vi "DB- Part setting.vi"(5 "string":string="Where partno='", 6 "Enum":T2(ring), 7 "Data Insert":variant, 8 "error in (no error)":errorcluster, 9 "columnsName":string[](array[string]), 10 "Model Name":string, 11 "connection reference":T1) -> (0 "error out":errorcluster, 2 "Data Read":variant[][](array[variant]), 3 "Refnum out":T1)   [LabVIEW 2015]
uses:
  <vilib>/addons/database/Connection.llb/Conn ObjectReference.ctl
  <vilib>/addons/database/NI_Database_API.lvlib
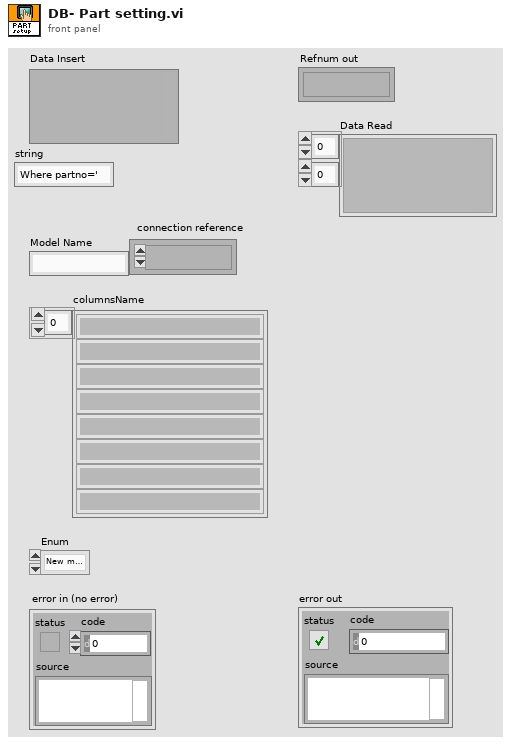
[diagram p1: front panel]
types:
  T1 = typedef "NI_Database_API.lvlib/Conn ObjectReference.ctl" = refnum<k1>
  T2 = enum16{"New model Create", "Update", "DB-Read by condition", "DB-Read", "Delete"}
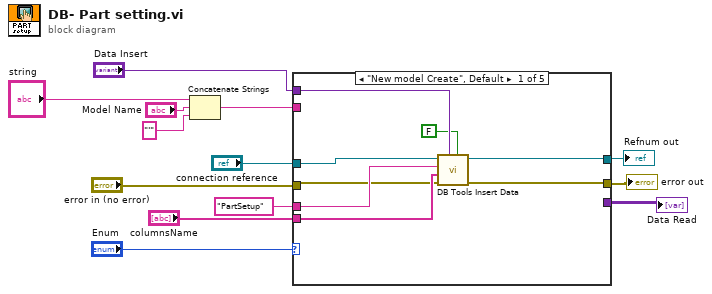
[diagram p0: block diagram]
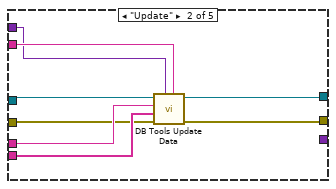
[diagram p2: hidden frame]
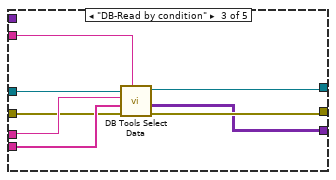
[diagram p3: hidden frame]
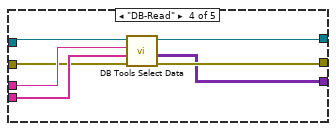
[diagram p4: hidden frame]
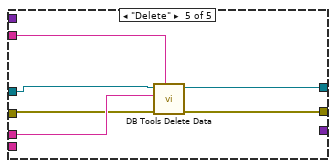
[diagram p5: hidden frame]
diagram:
  n1 = Concatenate Strings("string", "Model Name", "'" ("string")) -> (w9:string)
  n2 = case shown="\"New model Create\", Default" "Enum" {
    tunnel: [w21 w29 w34 w44 w50] -> w4
    tunnel: [w20 w28 w33 w43 w49] -> w5
    tunnel: w9 -> [_ w27 w37 _ w48]
    tunnel: "columnsName" -> [w19 w26 w36 w40 _]
    tunnel: "PartSetup" ("table") -> [w18 w25 w35 w41 w47]
    tunnel: "Data Insert" -> [w17 w24 _ _ _]
    tunnel: [_ _ w32 w42 _] -> w13
    tunnel: "connection reference" -> [w16 w23 w31 w39 w46]
    tunnel: "error in (no error)" -> [w15 w22 w30 w38 w45]
    frame "New model Create", Default {
      n3 = call <vilib>:"DB Tools Insert Data.vi"("create table? (F)"=FALSE, "data"=w17, "error in (no error)"=w15, "columns"=w19, "table"=w18, "connection reference"=w16) -> ("error out"=w20:errorcluster, "connection reference out"=w21:T1)  [unwired: 4 in]
    }
    frame "Update" {
      n4 = call <vilib>:"DB Tools Update Data.vi"("condition"=w27, "data"=w24, "error in (no error)"=w22, "columns"=w26, "table"=w25, "connection reference"=w23) -> ("error out"=w28:errorcluster, "connection reference out"=w29:T1)  [unwired: 4 in]
    }
    frame "DB-Read by condition" {
      n5 = call <vilib>:"DB Tools Select Data.vi"("condition"=w37, "error in (no error)"=w30, "columns"=w36, "table"=w35, "connection reference"=w31) -> ("error out"=w33:errorcluster, "data"=w32:variant[][], "connection reference out"=w34:T1)  [unwired: 1 in]
    }
    frame "DB-Read" {
      n6 = call <vilib>:"DB Tools Select Data.vi"("error in (no error)"=w38, "columns"=w40, "table"=w41, "connection reference"=w39) -> ("error out"=w43:errorcluster, "data"=w42:variant[][], "connection reference out"=w44:T1)  [unwired: 2 in]
    }
    frame "Delete" {
      n7 = call <vilib>:"DB Tools Delete Data.vi"("condition"=w48, "error in (no error)"=w45, "table"=w47, "connection reference"=w46) -> ("error out"=w49:errorcluster, "connection reference out"=w50:T1)  [unwired: 6 in]
    }
  }
  "Refnum out" <- w4
  "error out" <- w5
  "Data Read" <- w13
